vi "301_Module-DAQ_introduction_Single.vi"() -> ()   [LabVIEW 2009]
uses:
  <instrlib>/Zurich Instruments LabOne/Public/Modules/ziTypeModEnum.ctl
  <instrlib>/Zurich Instruments LabOne/Public/Modules/ziModSetValueDoubleArray.vi
  <instrlib>/Zurich Instruments LabOne/Public/Modules/ziModSetValueBinary.vi
  <instrlib>/Zurich Instruments LabOne/Public/Utility/ziTicksToS_vector.vi
  <instrlib>/Zurich Instruments LabOne/Public/Modules/ziModGetDoubleData.vi
  <instrlib>/Zurich Instruments LabOne/Zurich Instruments LabOne.lvlib
panel:
  out "XY Graph":cluster{"Timestamp(s)":dbl[], "Value":dbl[]}[](graph)
  in  "Columns":i32=10 caption="Number of Points"
  in  "Duration":dbl=1.0
  out "Connected?":bool
  out "Error Out":errorcluster
  in  "Address":string="DEV"
  # "LabOne Modules - DAQ introduction\nThis VI shows how to configure the DAQ module and capture lock-in data. It runs the DAQ module once to capture a defined number of points spanned over a defined duration given in seconds.\n\nSee block diagram for the VI description.\n\nRequirements: A Zurich Instrument lock-in amplifier\n\nTo run\n1- Type the Instrument ID\n2- Set the sampling duration and number of points.  \n3- Run the VI. It will turn on the signal output of the instrument.\n* You can change Node1 and Value1 Set in the back panel to set different nodes \n\nTested Devices:\n- HF2LI\n- UHFLI\n- MFLI\n\n(c) Zurich Instruments.  ALL RIGHTS RESERVED."
  # "For this VI to work you need to enable the data transfer of the first demodulator in the LabOne user interface"
  # "The Lock-in panel of your instrument might slightly differ depending on the instrument \nand installed options"
  # "The Lock-in panel of your instrument might slightly differ depending on the instrument \nand installed options"
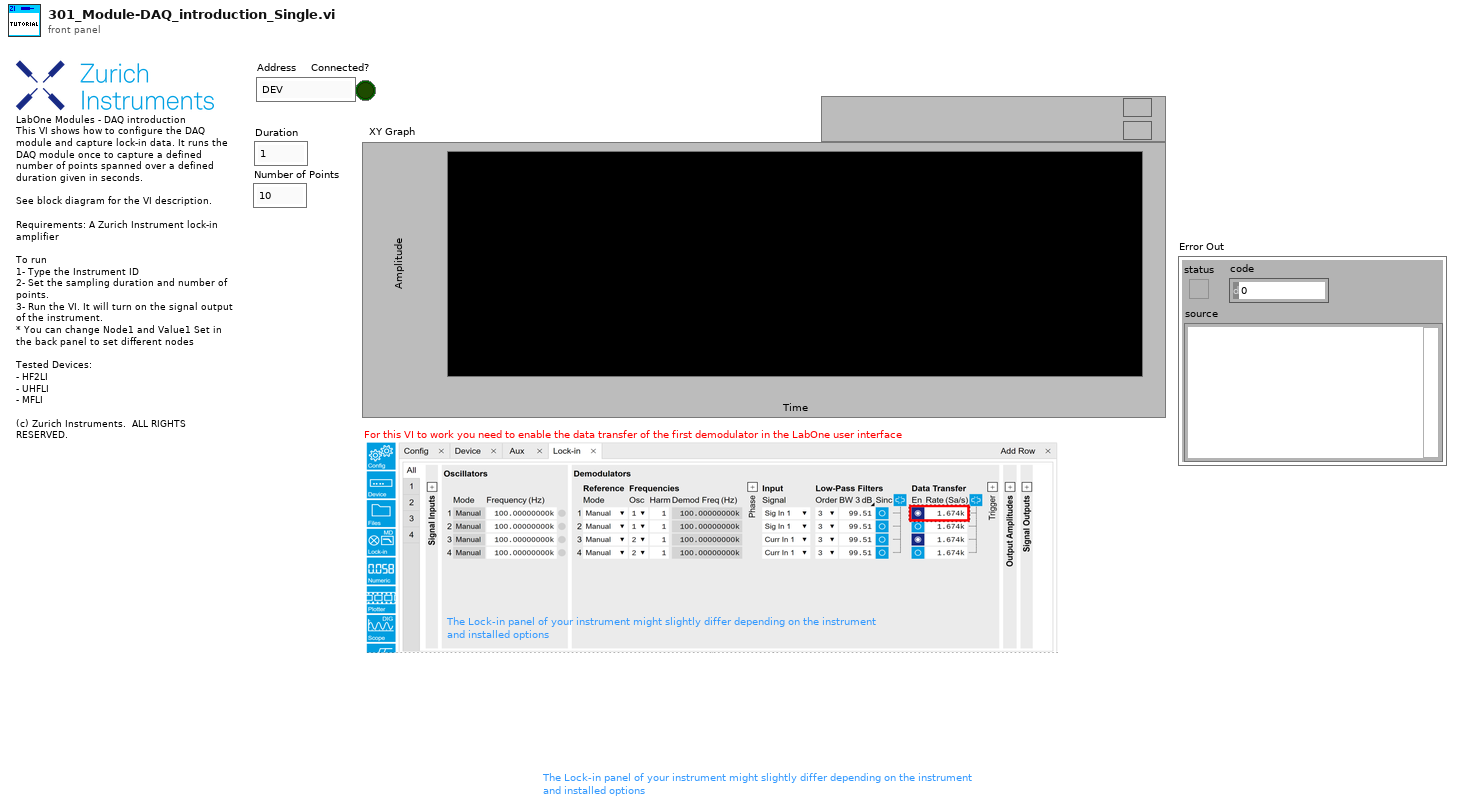
[diagram p1: front panel]
types:
  T1 = cluster{"path":string[], "Value":dbl[][], "Elapsed time (s)":dbl[][]}
  T2 = typedef "Zurich Instruments LabOne.lvlib/ziTypeModEnum.ctl" = u16
  T3 = typedef "Zurich Instruments LabOne.lvlib/ziTypeHandle.ctl" = cluster{"handleValid":bool, "Conn":u64, "Path Prefix":string, "Handle":u64, "Connected":bool, "Clockbase(s)":dbl}
  T4 = typedef "Zurich Instruments LabOne.lvlib/ziTypeModHandle.ctl" = cluster{"handleValid":bool, "Conn":u64, "ModHandle":u64, "moduleID":string, "Path Prefix":string}
  T5 = typedef "Zurich Instruments LabOne.lvlib/ziTypeModResults.ctl" = cluster{"PathArray":string[], "ValueType":T6, "NoOfResults":u64, "ziGenericHeader":T7[]}
  T6 = typedef "Zurich Instruments LabOne.lvlib/ziTypePollType.ctl" = enum16{"NONE", "DOUBLE_DATA", "INTEGER_DATA", "DEMOD_SAMPLE", "SCOPE_WAVE_HF2", "AUXIN_SAMPLE", "DIO_SAMPLE", "BYTE_ARRAY", "PWA_WAVE", "9", "10", "11", "12", "13", "14", "15", "TREE_CHANGE_DEPRI", "17", "ERROR", "19", "20", "21", "22", "23", "24", "25", "26", "27", "28", "29", "30", "31", "DOUBLE_DATA_TS", "INTEGER_DATA_TS", "34", "SCOPE_WAVE", "SCOPE_WAVE_EX", "37", "BYTE_ARRAY_TS", "39", "40", "41", "42", "43", "44", "45", "CNT_DATA", "47", "TREE_CHANGE", "49", "50", "51", "52", "53", "54", "55", "56", "57", "58", "59", "60", "61", "62", "63", "SWEEPER_DATA", "SPECTRUM_DATA", "ADVISOR_DATA", "VECTOR_DATA", "IMP_DATA", "SHF_GENERATOR_WAVEFORM_DATA", "SHF_RESULT_LOGGER_DATA", "SHF_SCOPE_DATA", "DEMOD_VECTOR"}
  T7 = typedef "Zurich Instruments LabOne.lvlib/ziTypeModGenericHeader.ctl" = cluster{"HeaderType":enum8{"HEADER_TYPE_NONE", "HEADER_TYPE_SWTRIGGER", "HEADER_TYPE_SWEEPER"}, "SampleFormat":u8, "SystemTime":timestamp, "CreatedTimeStamp":u64, "ChangedTimeStamp":u64, "Flags":u32, "ChunkSizeBytes":u64, "Name":string, "Status":u32, "GroupIndex":u32, "Color":u32, "ActiveRow":u32, "TriggerNumber":u64, "GridRows":u32, "GridCols":u32, "GridMode":u32, "GridOperation":u32, "GridDirection":u32, "GridRepetitions":u32, "GridColDelta":dbl, "GridColOffset":dbl, "GridRowDelta":dbl, "GridRowOffset":dbl, "Bandwidth":dbl, "Center":dbl, "Nenbw":dbl}
  T8 = typedef "Zurich Instruments LabOne.lvlib/ziTypeDoubleDataTS.ctl" = cluster{"Timestamp (ticks)":u64[], "Value":dbl[]}
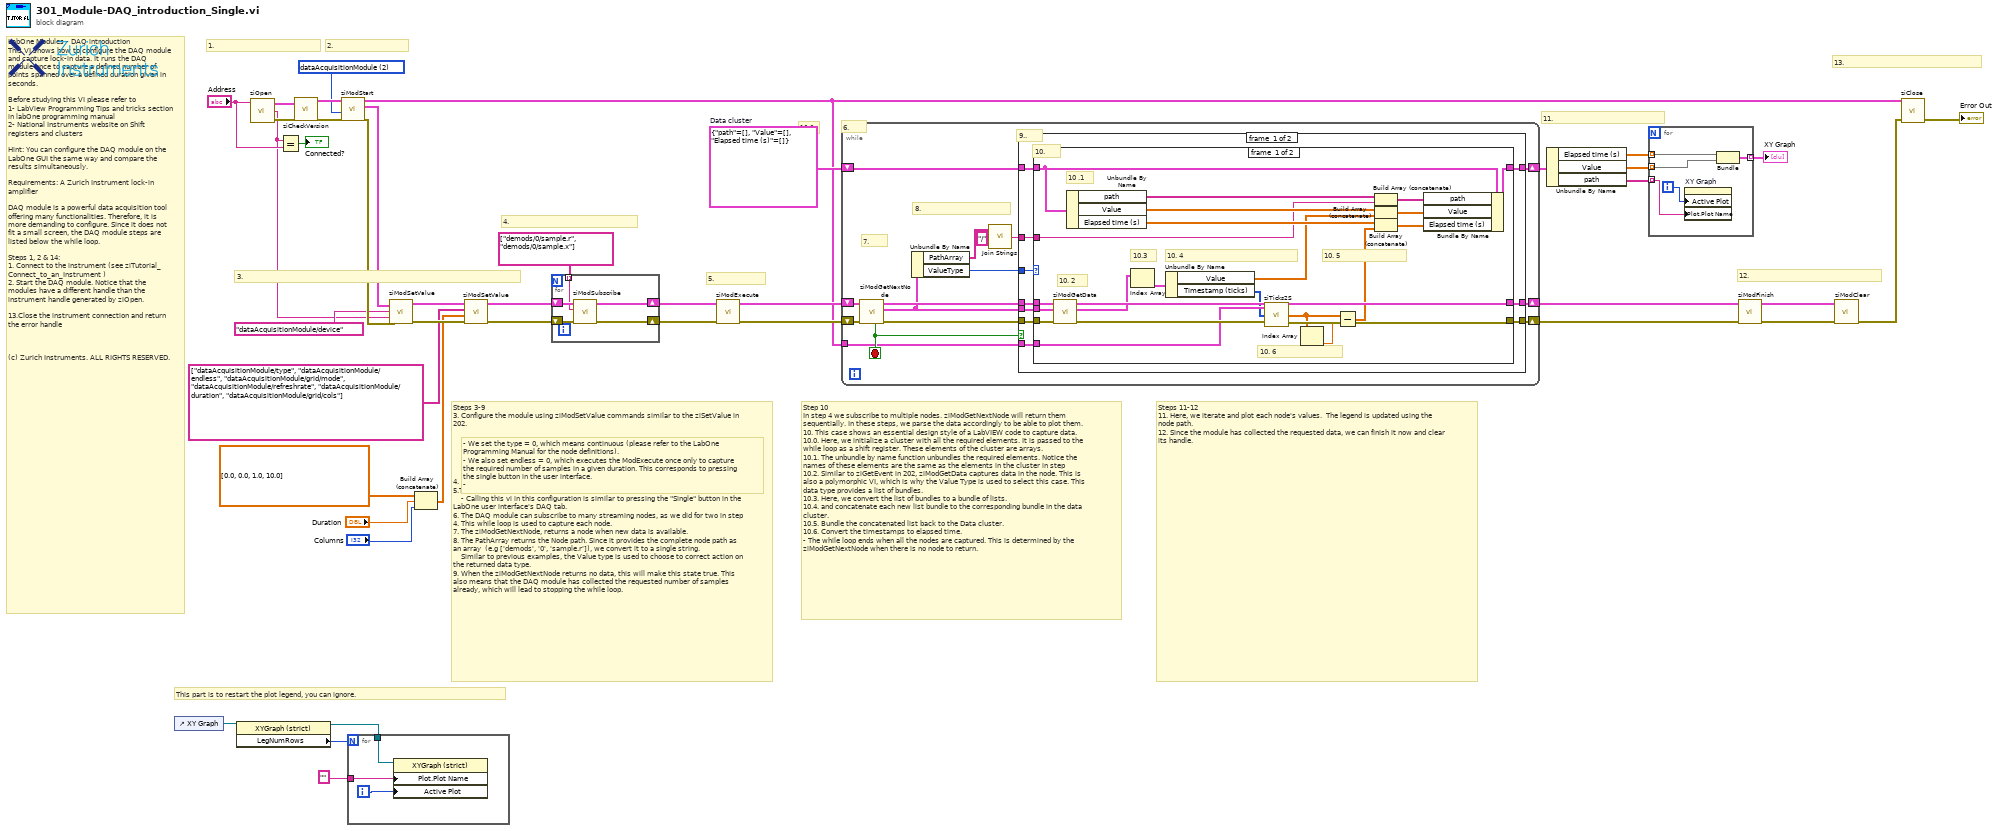
[diagram p0: block diagram]
diagram:
  w13 = T1 {"path"=[], "Value"=[], "Elapsed time (s)"=[]}  # Data cluster
  w35 = T2 2 items=["sweep", "scopeModule", "dataAcquisitionModule", "pidAdvisor", "awgModule", "impedanceModule", "multiDeviceSyncModule", "zoomFFT", "trigger", "deviceSettings", "record"] ("module Id")
  # "- We set the type = 0, which means continuous (please refer to the LabOne Programming Manual for the node definitions). \n- We also set endless = 0, which executes the ModExecute once only to capture the required number of samples in a given duration. This corresponds to pressing the single button in the user interface.\n-"
  # "6."
  # "5."
  # "11."
  # "12."
  # "10.0."
  # "This part is to restart the plot legend, you can ignore."
  # "Steps 11-12\n11. Here, we iterate and plot each node's values.  The legend is updated using the node path.\n12. Since the module has collected the requested data, we can finish it now and clear its handle."
  # "Step 10\nIn step 4 we subscribe to multiple nodes. ziModGetNextNode will return them sequentially. In these steps, we parse the data accordingly to be able to plot them.\n10. This case shows an essential design style of a LabVIEW code to capture data.\n10.0. Here, we initialize a cluster with all the required elements. It is passed to the while loop as a shift register. These elements of the cluster are arrays.\n10.1. The unbundle by name function unbundles the required elements. Notice the names of these elements are the same as the elements in the cluster in step \n10.2. Similar to ziGetEvent in 202, ziModGetData captures data in the node. This is also a polymorphic VI, which is why the Value Type is used to select this case. This data type provides a list of bundles. \n10.3. Here, we convert the list of bundles to a bundle of lists.\n10.4. and concatenate each new list bundle to the corresponding bundle in the data cluster.\n10.5. Bundle the concatenated list back to the Data cluster.\n10.6. Convert the timestamps to elapsed time.\n- The while loop ends when all the nodes are captured. This is determined by the ziModGetNextNode when there is no node to return."
  # "Steps 3-9\n3. Configure the module using ziModSetValue commands similar to the ziSetValue in 202. \n\n\n\n\n\n\n4. Subscribe to the nodes that we intend to capture.2\n5.The module starts to operate after the ziModExecute command. \n    - Calling this vi in this configuration is similar to pressing the \"Single\" button in the LabOne user interface's DAQ tab.\n6. The DAQ module can subscribe to many streaming nodes, as we did for two in step 4. This while loop is used to capture each node. \n7. The ziModGetNextNode, returns a node when new data is available.\n8. The PathArray returns the Node path. Since it provides the complete node path as an array  (e.g ['demods', '0', 'sample.r']), we convert it to a single string. \n    Similar to previous examples, the Value type is used to choose to correct action on the returned data type. \n9. When the ziModGetNextNode returns no data, this will make this state true. This also means that the DAQ module has collected the requested number of samples already, which will lead to stopping the while loop."
  # "4."
  # "3."
  # "2."
  # "1."
  # "13."
  # "LabOne Modules - DAQ introduction\nThis VI shows how to configure the DAQ module and capture lock-in data. It runs the DAQ module once to capture a defined number of points spanned over a defined duration given in seconds.\n\nBefore studying this VI please refer to \n1- LabView Programming Tips and tricks section in labOne programming manual\n2- National Instruments website on Shift registers and clusters\n\nHint: You can configure the DAQ module on the LabOne GUI the same way and compare the results simultaneously. \n\nRequirements: A Zurich Instrument lock-in amplifier\n\nDAQ module is a powerful data acquisition tool offering many functionalities. Therefore, it is more demanding to configure. Since it does not fit a small screen, the DAQ module steps are listed below the while loop. \n\nSteps 1, 2 & 14:\n1. Connect to the instrument (see ziTutorial_Connect_to_an_Instrument )\n2. Start the DAQ module. Notice that the modules have a different handle than the instrument handle generated by ziOpen. \n\n13.Close the instrument connection and return the error handle   \n\n\n\n(c) Zurich Instruments. ALL RIGHTS RESERVED."
  n1 = control-ref of="XY Graph"() -> (w17:refnum<vi>)
  n2 = property class="XYGraph (strict)"(reference=w17) -> (reference out=w15:refnum<vi>, "LegNumRows"=w16:u32)  [unwired: 1 in, 1 out]
  n3 = call <instrlib>:"ziOpen.vi"("Address"="Address") -> ("Error Out"=w38:errorcluster, "Selected Device"=w31:string, "HandleOut"=w39:T3)  [unwired: 1 in, 2 out]
  n4 = Equal?(x=w31, y="Address") -> (x = y?=→"Connected?":bool)
  n5 = call <instrlib>:"ziCheckVersion.vi"("Handle In"=w39, "Error In"=w38) -> ("Handle Out"=w36:T3, "Error Out"=w37:errorcluster)  [unwired: 11 in, 1 out]
  n6 = call <instrlib>:"ziModStart.vi"("Error In"=w37, "module Id"=w35, "Handle In"=w36) -> ("Error Out"=w33:errorcluster, "ModHandle Out"=w34:T4, "Handle Out"=w3:T3)  [unwired: 6 in]
  n7 = for {
    N: w16 -> [_]
    tunnel: w15 -> [w45]
    tunnel: "" -> [w44]
    i -> [w43]
    n8 = property class="XYGraph (strict)"(reference=w45, "Plot.Plot Name"=w44, "Active Plot"=w43) -> ()  [unwired: 1 in, 2 out]
  }
  n9 = call-poly <instrlib>:"ziModSetValue.vi"("Error In"=w33, "Data"=w31, "Path"="dataAcquisitionModule/device", "ModHandle In"=w34) -> ("Error Out"=w29:errorcluster, "ModHandle Out"=w30:T4)  [unwired: 6 in]
  n10 = Build Array (concatenate)(dbl[] [0.0, 0.0, 1.0, 10.0], "Duration", "Columns") -> (w26:dbl[])
  n11 = call-poly <instrlib>:"ziModSetValue.vi"("Error In"=w29, "Values"=w26, "Paths"=string[] ["dataAcquisitionModule/type", "dataAcquisitionModule/endless", "dataAcquisitionModule/grid/mode", "dataAcquisitionModule/refreshrate", "dataAcquisitionModule/duration", "dataAcquisitionModule/grid/cols"], "ModHandle In"=w30) -> ("Error Out"=w19:errorcluster, "ModHandle Out"=w20:T4)  [unwired: 6 in]
  n12 = for {
    shift-right: [w50] -> w22
    shift-left: w20 -> [w48]
    shift-right: [w49] -> w21
    shift-left: w19 -> [w47]
    tunnel: string[] ["demods/0/sample.r", "demods/0/sample.x"] -> [w46] mode=indexing
    n13 = call <instrlib>:"ziModSubscribe.vi"("Error In"=w47, "Path"=w46, "ModHandle In"=w48) -> ("Error Out"=w49:errorcluster, "ModHandle Out"=w50:T4)  [unwired: 6 in]
  }
  n14 = call <instrlib>:"ziModExecute.vi"("Error In"=w21, "ziModHandle In"=w22) -> ("Error Out"=w4:errorcluster, "ziModHandle Out"=w5:T4)  [unwired: 7 in]
  n15 = while {
    shift-right: [w57] -> w10
    shift-left: w13 -> [w58]
    shift-right: [w52] -> w11
    shift-left: w5 -> [w64]
    shift-right: [w53] -> w12
    shift-left: w4 -> [w65]
    tunnel: w3 -> [w51]
    stop <- w63 stop-if-true
    # "9.."
    # "8."
    # "7."
    n16 = call <instrlib>:"ziModGetNextNode.vi"("Error In"=w65, "ModHandle In"=w64) -> ("Error Out"=w62:errorcluster, "ModResults"=w60:T5, "ModHandle Out"=w61:T4, "NoData"=w63:bool)  [unwired: 6 in]
    n17 = Unbundle By Name(w60) -> ("PathArray"=w55:string[], "ValueType"=w59:T6)
    n18 = call <vilib>:"Join Strings.vi"("Separator (,)"="/", "Strings In"=w55) -> ("String"=w54:string)  [unwired: 1 in]
    n19 = case shown="False" w63 {
      tunnel: w62 -> [w73 w103]
      tunnel: w61 -> [w74 w104]
      tunnel: [w71 w104] -> w52
      tunnel: [w72 w103] -> w53
      tunnel: w60 -> [w75 _]
      tunnel: w59 -> [w70 _]
      tunnel: [w69 w102] -> w57
      tunnel: w58 -> [w68 w102]
      tunnel: w54 -> [w67 _]
      tunnel: w51 -> [w66 _]
      frame #0 {
        # "10."
        n20 = case shown="\"DOUBLE_DATA_TS\"" w70 {
          tunnel: w75 -> [w98 _]
          tunnel: w74 -> [w97 w100]
          tunnel: w73 -> [w96 w99]
          tunnel: [w81 w99] -> w72
          tunnel: [w95 w100] -> w71
          tunnel: [w91 w101] -> w69
          tunnel: w68 -> [w92 w101]
          tunnel: w67 -> [w84 _]
          tunnel: w66 -> [w80 _]
          frame #0 {
            # "10. 6"
            # "10. 5"
            # "10. 4"
            # "10.3"
            # "10. 2"
            # "10 .1"
            n21 = call-poly <instrlib>:"ziModGetData.vi"("Error In"=w96, "ModResults"=w98, "ModHandle In"=w97) -> ("Error Out"=w82:errorcluster, "DoubleSample"=w94:T8[], "ModHandle Out"=w95:T4)  [unwired: 4 in, 2 out]
            n22 = Unbundle By Name(w92) -> ("path"=w90:string[], "Value"=w88:dbl[][], "Elapsed time (s)"=w85:dbl[][])
            n23 = Index Array(array=w94) -> (element=w93:T8)  [unwired: 1 in]
            n24 = Unbundle By Name(w93) -> ("Value"=w83:dbl[], "Timestamp (ticks)"=w79:u64[])
            n25 = call-poly <instrlib>:"ziTicks2S.vi"("Error In"=w82, "Timestamp (ticks)"=w79, "Handle In"=w80) -> ("Error Out"=w81:errorcluster, "Timestamp(s)"=w78:dbl[])  [unwired: 1 out]
            n26 = Index Array(array=w78) -> (element=w77:dbl)  [unwired: 1 in]
            n27 = Subtract(x=w78, y=w77) -> (x-y=w76:dbl[])
            n28 = Build Array (concatenate)(w90, w84) -> (w89:string[])
            n29 = Build Array (concatenate)(w88, w83) -> (w87:dbl[][])
            n30 = Build Array (concatenate)(w85, w76) -> (w86:dbl[][])
            n31 = Bundle By Name(cluster=w92, "path"=w89, "Value"=w87, "Elapsed time (s)"=w86) -> (w91:T1)
          }
          frame #1 {
          }
        }
      }
      frame #1 {
      }
    }
  }
  n32 = Unbundle By Name(w10) -> ("Elapsed time (s)"=w9:dbl[][], "Value"=w8:dbl[][], "path"=w6:string[])
  n33 = for {
    tunnel: w9 -> [w107] mode=indexing
    tunnel: w8 -> [w109] mode=indexing
    tunnel: [w108] -> w7 mode=indexing
    tunnel: w6 -> [w106] mode=indexing
    i -> [w105]
    n34 = property on="XY Graph" class="XYGraph (strict)"("Active Plot"=w105, "Plot.Plot Name"=w106) -> ()  [unwired: 2 in, 2 out]
    n35 = Bundle("Elapsed time (s)"=w107, "Value"=w109) -> (w108:cluster{"Elapsed time (s)":dbl[], "Value":dbl[]})  [unwired: 1 in]
  }
  "XY Graph" <- w7
  n36 = call <instrlib>:"ziModFinish.vi"("Error In"=w12, "ziModHandle In"=w11) -> ("Error Out"=w25:errorcluster, "ziModHandle Out"=w24:T4)  [unwired: 7 in]
  n37 = call <instrlib>:"ziModClear.vi"("Error In"=w25, "ziModHandle In"=w24) -> ("Error Out"=w23:errorcluster)  [unwired: 7 in, 1 out]
  n38 = call <instrlib>:"ziClose.vi"("Error In"=w23, "Handle In"=w3) -> ("Error Out"=→"Error Out":errorcluster)  [unwired: 2 in, 1 out]
